vi "array_last_elmt_test.vi"() -> ()   [LabVIEW 2010]
panel:
  out "Value":dbl
  in  "Array":dbl[](array[numeric])
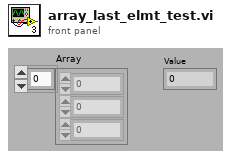
[diagram p1: front panel]
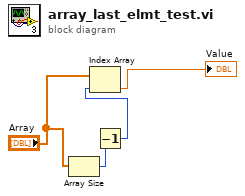
[diagram p0: block diagram]
diagram:
  n1 = Array Size(array="Array") -> (size(s)=w2:i32)
  n2 = Decrement(x=w2) -> (x-1=w1:i32)
  n3 = Index Array(array="Array", index=w1) -> (element=→"Value":dbl)
